vi "指定多时刻（时分秒）闹钟.vi"(8 "Error In":errorcluster caption="错误输入", 9 "模式":enum16{"秒", "分", "时"}(ring), 10 "偏移量":i32[](array[numeric])) -> (0 "Error Out":errorcluster caption="错误输出", 1 "时刻":i32, 3 "时间到":bool)   [LabVIEW 2012]
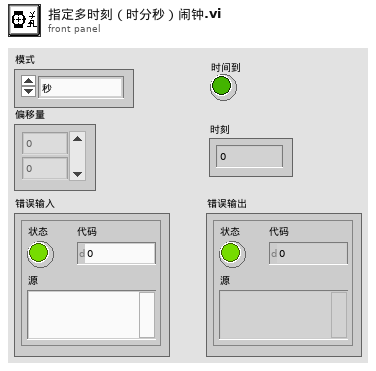
[diagram p1: front panel]
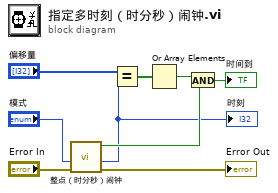
[diagram p0: block diagram]
diagram:
  n1 = call "整点（时分秒）闹钟.vi"("Error In"="Error In", "模式"="模式") -> ("Error Out"=→"Error Out":errorcluster, "时刻"=w3:i32, "时间到"=w5:bool)  [unwired: 7 in]
  "时刻" <- w3
  n2 = Equal?(x="偏移量", y=w3) -> (x = y?=w2:bool[])
  n3 = Or Array Elements(Boolean array=w2) -> (logical OR=w1:bool)
  n4 = And(x=w1, y=w5) -> (x .and. y?=→"时间到":bool)
